vi "DFD NStage MRate Filtering (Wfm).vi"(6 "zero phase? (T)":bool=TRUE, 7 "init? (F)":bool, 8 "error in (no error)":errorcluster, 10 "multirate filters":T1[](array[typedef]) {"mMRate_SumWl" min=1 max=32 step=1; "mMRate_InputIwl" min=1 max=32 step=1; "mMRate_GainWl" min=1 max=32 step=1; "mMRate_OutputWl" min=1 max=32 step=1; "mMRate_InputWl" min=1 max=32 step=1; "mMRate_CoefWl" min=1 max=32 step=1; "mMRate_Mode" items=["Default"=-1, "No Rate Change"=0, "Interpolation"=1, "Decimation"=2, "Interpolated"=3, "Rational"=4]}, 11 "signal in":waveform(dbl)={"t0"=timestamp(0 s since 1904-01-01), "dt"=0.0, "Y"=[]}) -> (0 "error out":errorcluster, 3 "signal out":waveform(dbl))   [LabVIEW 2017, in "NI_DigFilterLicensed.lvlib"]
doc: "Filters a signal continuously with a multistage multirate filter. Wire data to the <B>signal in</B> input to determine the polymorphic instance to use or manually select the instance."
uses:
  <vilib>/addons/Digital Filter Design/NI_DigFilterLicensed.lvlib
  <vilib>/addons/Digital Filter Design/_Objects.llb/DFD Multirate Filter Obj.ctl
  <vilib>/addons/Digital Filter Design/_Objects.llb/DFD Multirate Mode.ctl
  <vilib>/addons/Digital Filter Design/_Objects.llb/DFD Coef Norm Type.ctl
  <vilib>/addons/Digital Filter Design/_Objects.llb/DFD Round-off Mode.ctl
  <vilib>/addons/Digital Filter Design/_Objects.llb/DFD FXP MRate Multiply Mode.ctl
  <vilib>/addons/Digital Filter Design/NI_DigFilter_Process.lvlib
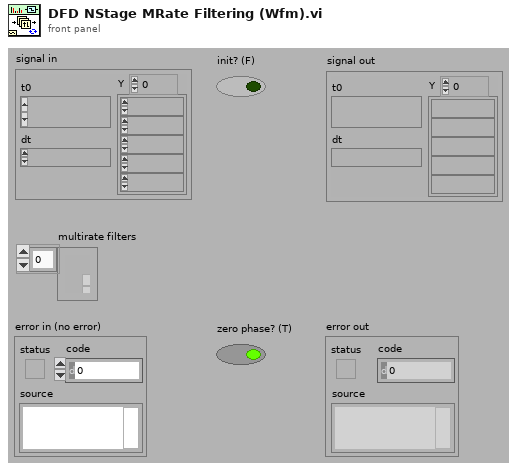
[diagram p1: front panel]
types:
  T1 = typedef "NI_DigFilterLicensed.lvlib/DFD Multirate Filter Obj.ctl" = cluster{"mMRate_Structure":enum16{"CIC", "FIR", "IIR", "Lattice"}, "mMRate_Mode":T2, "mMRate_Factor":i32, "mMRate_FIRParams":cluster{"mMRate_FIR_H":dbl[], "mMRate_FIR_IsNyquist?":bool, "mMRate_FIR_IsSymmetric?":bool}, "mMRate_CICParams":cluster{"mMRate_CIC_#Stage":i32, "mMRate_CIC_Lag":i32, "mMRate_CIC_Type":enum16{"Lowpass", "Highpass"}}, "mMRate_Order":i32, "mMRate_Version":string, "mMRate_Comments":string, "mMRate_RationalFactor":cluster{"mMRate_L":i32, "mMRate_M":i32}, "mMRate_Fs":dbl, "mMRate_Quantized?":bool, "mMRate_QFilterGain":dbl, "mMRate_CoefWl":i16, "mMRate_Scaling":cluster{"mMRate_ScaleByPowerOf2?":bool, "mMRate_ScaleType":T3}, "mMRate_InputWl":i16, "mMRate_OutputWl":i16, "mMRate_OutputMode":T4, "mMRate_MultMode":T5, "mMRate_BitPruning":bool, "mMRate_GainWl":i16, "mMRate_OutputFwl":i16, "mMRate_SumIwl":i16, "mMRate_InputIwl ":i16, "mMRate_SumWl":i16, "mMRate_CoefIwl":i16}
  T2 = typedef "NI_DigFilterLicensed.lvlib/DFD Multirate Mode.ctl" = i16
  T3 = typedef "NI_DigFilterLicensed.lvlib/DFD Coef Norm Type.ctl" = enum16{"No Norm", "Time Domain 1-Norm", "Time Domain 2-Norm", "Time Domain Inf-Norm"}
  T4 = typedef "NI_DigFilterLicensed.lvlib/DFD Round-off Mode.ctl" = enum16{"Nearest", "Truncation"}
  T5 = typedef "NI_DigFilterLicensed.lvlib/DFD FXP MRate Multiply Mode.ctl" = enum16{"Truncated", "Full"}
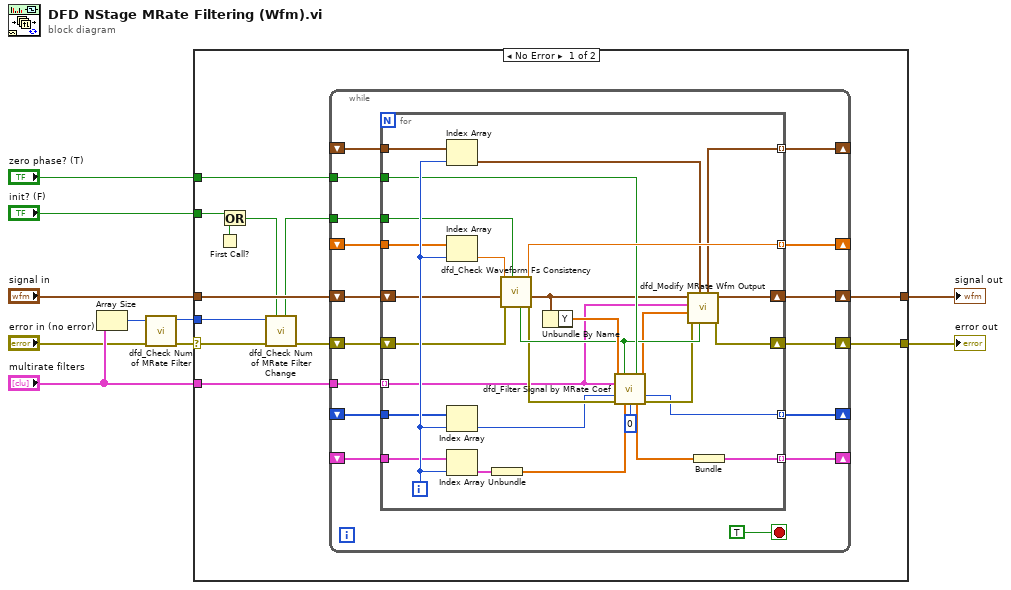
[diagram p0: block diagram]
diagram:
  n1 = Array Size(array="multirate filters") -> (size(s)=w3:i32)
  n2 = call <vilib>:"dfd_Check Num of MRate Filter.vi"("error in (no error)"="error in (no error)", "#MRate in"=w3) -> ("error out"=w1:errorcluster, "#MRate out"=w2:i32)  [unwired: 8 out]
  n3 = case shown="No Error" w1 {
    selector: w1 -> [w18 w68]
    tunnel: [w12 w68] -> w8
    tunnel: "multirate filters" -> [w17 _]
    tunnel: "signal in" -> [w19 _]
    tunnel: [w13 _] -> w10
    tunnel: "zero phase? (T)" -> [w20 _]
    tunnel: "init? (F)" -> [w21 _]
    tunnel: w2 -> [w11 _]
    frame No Error {
      n4 = First Call?() -> (First Call?: T/F=w22:bool)
      n5 = Or(x=w21, y=w22) -> (x .or. y?=w15:bool)
      n6 = call <vilib>:"dfd_Check Num of MRate Filter Change.vi"("init in"=w15, "error in (no error)"=w18, "#MRate in"=w11) -> ("error out"=w16:errorcluster, "init out"=w14:bool)  [unwired: 7 out]
      n7 = while {
        shift-right: [w23] -> _
        shift-left: _ -> [w33]
        tunnel: w14 -> [w28]
        shift-right: [w27] -> _
        shift-left: _ -> [w36]
        shift-right: [w29] -> _
        shift-left: _ -> [w35]
        tunnel: w20 -> [w31]
        shift-right: [w24] -> _
        shift-left: _ -> [w34]
        shift-right: [w26] -> w13
        shift-left: w19 -> [w38]
        tunnel: w17 -> [w25]
        shift-right: [w32] -> w12
        shift-left: w16 -> [w30]
        stop <- TRUE stop-if-true
        n8 = for {
          tunnel: w33 -> [w43]
          tunnel: w36 -> [w56]
          shift-right: [w49] -> w32
          shift-left: w30 -> [w52]
          tunnel: w35 -> [w65]
          tunnel: w34 -> [w47]
          tunnel: w31 -> [w60]
          tunnel: [w63] -> w29 mode=indexing
          tunnel: w28 -> [w62]
          tunnel: [w54] -> w27 mode=indexing
          tunnel: w25 -> [w48] mode=indexing
          tunnel: [w46] -> w24 mode=indexing
          tunnel: [w41] -> w23 mode=indexing
          shift-right: [w53] -> w26
          shift-left: w38 -> [w66]
          i -> [w67]
          n9 = Index Array(array=w56, index=w67) -> (element=w55:timestamp)
          n10 = Index Array(array=w65, index=w67) -> (element=w64:dbl)
          n11 = Index Array(array=w47, index=w67) -> (element=w45:i32)
          n12 = Index Array(array=w43, index=w67) -> (element=w40:cluster{"state out":dbl[]})
          n13 = Unbundle(w40) -> ("state out"=w39:dbl[])
          n14 = call <vilib>:"dfd_Check Waveform Fs Consistency.vi"("init in"=w62, "error in (no error)"=w52, "signal in"=w66, "dt in"=w64) -> ("error out"=w51:errorcluster, "signal out"=w57:waveform(dbl), "dt out"=w63:dbl, "init out"=w59:bool)  [unwired: 4 out]
          n15 = Unbundle By Name(w57) -> ("Y"=w61:dbl[])
          n16 = call <vilib>:"dfd_Filter Signal by MRate Coef.vi"("signal in"=w61, "initH?"=w59, "zeroPhaseH?"=w60, "multirate filter"=w48, "skipPoint In"=w45, "error in (no error)"=w51, "state in"=w39, "outputPhase"=0) -> ("signal out"=w58:dbl[], "skipPoint Out"=w46:i32, "state out"=w44:dbl[], "error out"=w50:errorcluster)  [unwired: 4 out]
          n17 = call <vilib>:"dfd_Modify MRate Wfm Output.vi"("initH"=w59, "t0"=w55, "error in (no error)"=w50, "y"=w58, "multirate filter in"=w48, "x"=w57) -> ("error out"=w49:errorcluster, "y"=w53:waveform(dbl), "tf"=w54:timestamp)  [unwired: 3 out]
          n18 = Bundle("state out"=w44) -> (w41:cluster{"state out":dbl[]})  [unwired: 1 in]
        }
      }
    }
    frame Error {
    }
  }
  "error out" <- w8
  "signal out" <- w10
